vi "FinalStateNode_Create.vi"(0 "reference":refnum<class "FinalStateNode.lvclass">, 5 "error in (no error)":errorcluster) -> (14 "reference out":refnum<class "FinalStateNode.lvclass">, 19 "error out":errorcluster)   [LabVIEW 2020, in "FinalStateNode.lvclass"]
doc: "Creates and initializes a new FinalStateNode object.\n\nThis object should be destroyed using a FinalStateNode destructor VI or a virtual base class destructor VI.\n\n[GOOP 2.1]"
uses:
  <resource>/Framework/Providers/Open_GDS/UML/FinalStateNode_class/FinalStateNode.lvclass
  C:/Program Files (x86)/National Instruments/LabVIEW 2020/resource/Framework/Providers/Open_GDS/UML/RectangularNode_class/RectangularNode.lvclass
  <resource>/Framework/Providers/Open_GDS/UML/MultiLineString_class/SizeType.ctl
  <resource>/Framework/Providers/Open_GDS/UML/General/Rectangle/Rectangle Rectangle2D.ctl
  <resource>/Framework/Providers/Open_GDS/UML/MultiLineString_class/JustificationType.ctl
  <resource>/Framework/Providers/Open_GDS/UML/MultiLineString_class/MultiLineString.lvclass
  <resource>/Framework/Providers/Open_GDS/UML/RectangularNode_class/RectangularNode.lvclass
panel:
  # "The input reference should only\nbe wired when this method is called\nby a sub class constructor."
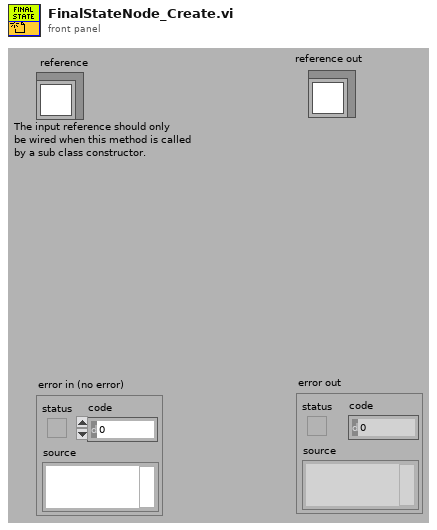
[diagram p1: front panel]
types:
  T1 = typedef "MultiLineString.lvclass/JustificationType.ctl" = enum16{"LEFT", "CENTER", "RIGHT"}
  T2 = typedef "Rectangle Rectangle2D.ctl" = cluster{"x":dbl, "y":dbl, "width":dbl, "height":dbl}
  T3 = typedef "MultiLineString.lvclass/SizeType.ctl" = enum16{"LARGE", "NORMAL", "SMALL"}
  T4 = typedef "FinalStateNode.lvclass/ObjectAttributes.ctl" = cluster{"name":refnum<class "MultiLineString.lvclass">, "DEFAULT_WIDTH":i32, "DEFAULT_HEIGHT":i32}
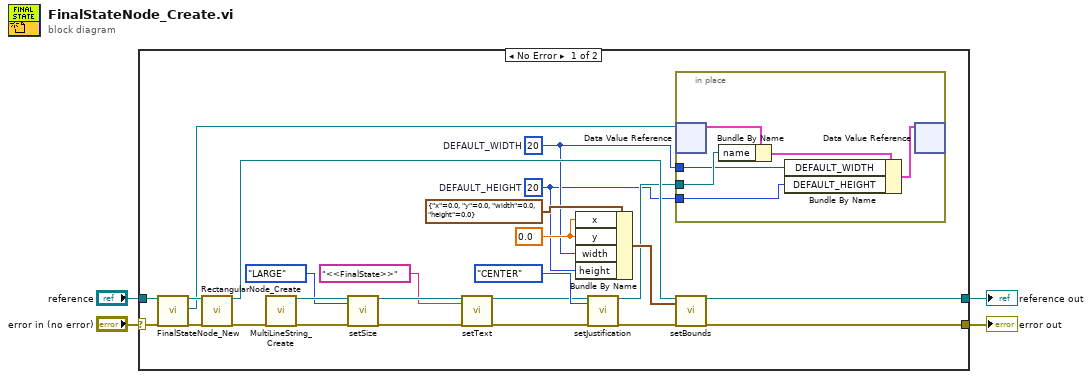
[diagram p0: block diagram]
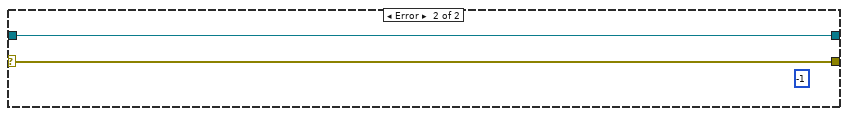
[diagram p2: hidden frame]
diagram:
  n1 = case shown="No Error" "error in (no error)" {
    selector: "error in (no error)" -> [w29 w37]
    tunnel: [w5 w36] -> w4
    tunnel: [w6 w37] -> w3
    tunnel: "reference" -> [w28 w36]
    frame No Error {
      w18 = 0.0 ("x")
      w8 = 20  # DEFAULT_HEIGHT
      w9 = 20  # DEFAULT_WIDTH
      n2 = call <resource>:"FinalStateNode_New.vi"("reference in"=w28, "error in (no error)"=w29) -> ("reference out"=w16:refnum<class "FinalStateNode.lvclass">, "DVRRefOut"=w7:refnum<data-value>, "error out"=w27:errorcluster)  [unwired: 2 in, 13 out]
      n3 = call <resource>:"RectangularNode_Create.vi"("reference"=w16, "error in (no error)"=w27) -> ("reference out"=w21:refnum<class "FinalStateNode.lvclass">, "error out"=w26:errorcluster)  [unwired: 1 in, 15 out]
      n4 = call <resource>:"MultiLineString_Create.vi"("error in (no error)"=w26) -> ("reference out"=w25:refnum<class "MultiLineString.lvclass">, "error out"=w24:errorcluster)  [unwired: 2 in, 15 out]
      n5 = call <resource>:"setSize.vi"("reference"=w25, "size"=SizeType."LARGE", "error in (no error)"=w24) -> ("reference out"=w15:refnum<class "MultiLineString.lvclass">, "error out"=w14:errorcluster)  [unwired: 15 out]
      n6 = call-dynamic "setText.vi"("reference"=w15, "text"="<<FinalState>>", "error in (no error)"=w14) -> ("reference out"=w11:refnum<class "MultiLineString.lvclass">, "error out"=w12:errorcluster)  [unwired: 15 in]
      n7 = Bundle By Name(cluster=T2 {"x"=0.0, "y"=0.0, "width"=0.0, "height"=0.0} ("bounds"), "x"=w18, "y"=w18, "width"=w9, "height"=w8) -> (w20:T2)
      n8 = call <resource>:"setJustification.vi"("reference"=w11, "justification"=JustificationType."CENTER", "error in (no error)"=w12) -> ("reference out"=w10:refnum<class "MultiLineString.lvclass">, "error out"=w17:errorcluster)  [unwired: 15 out]
      n9 = in-place {
        in-place-border: w10 -> [w34]
        in-place-border: w9 -> [w32]
        in-place-border: w8 -> [w31]
        n10 = in-place-dvr #1(w7) -> (w35:T4)  [unwired: 1 out]
        n11 = Bundle By Name(cluster=w35, "name"=w34) -> (w33:T4)
        n12 = Bundle By Name(cluster=w33, "DEFAULT_WIDTH"=w32, "DEFAULT_HEIGHT"=w31) -> (w30:T4)
        n13 = in-place-dvr #1(w30) -> ()  [unwired: 2 out]
      }
      n14 = call-dynamic "setBounds.vi"("reference"=w21, "bounds"=w20, "error in (no error)"=w17) -> ("reference out"=w5:refnum<class "FinalStateNode.lvclass">, "error out"=w6:errorcluster)  [unwired: 15 in]
    }
    frame Error {
      (unwired) -1 ("Nr of open handles")
    }
  }
  "error out" <- w3
  "reference out" <- w4
